vi "QuickRotation.vi"(7 "Á³±ì­±¦V":dbl(ring)=115.0 items=["Forward"=30.0, "Right"=120.0, "Left"=-65.0], 8 "Error In":errorcluster) -> (0 "Error Out":errorcluster)   [LabVIEW 2019]
uses:
  WSCbot_V3_Toolkit.lvlibp
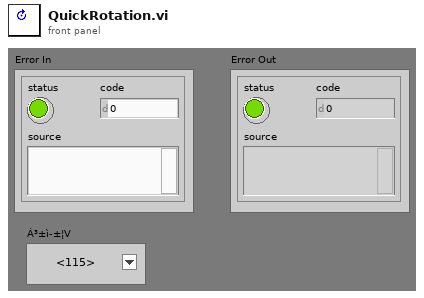
[diagram p1: front panel]
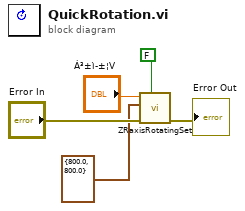
[diagram p0: block diagram]
diagram:
  n1 = call "ZRaxisRotatingSet.vi"("Reset"=FALSE, "error in"="Error In", "Velocity(deg/s)&ACC(deg/ss)"=cluster{"Velocity(cm/s)":dbl, "ACC(cm/ss)":dbl} {"Velocity(cm/s)"=800.0, "ACC(cm/ss)"=800.0}, "TargetHight(deg)"="Á³±ì­±¦V") -> ("error out"=→"Error Out":errorcluster)  [unwired: 6 in, 1 out]
